vi "DAQAssistantTests.vi"() -> ()   [LabVIEW 2017]
panel:
  out "Numeric":dbl
  out "XY Graph":cluster{dbl[], dbl[]}(graph)
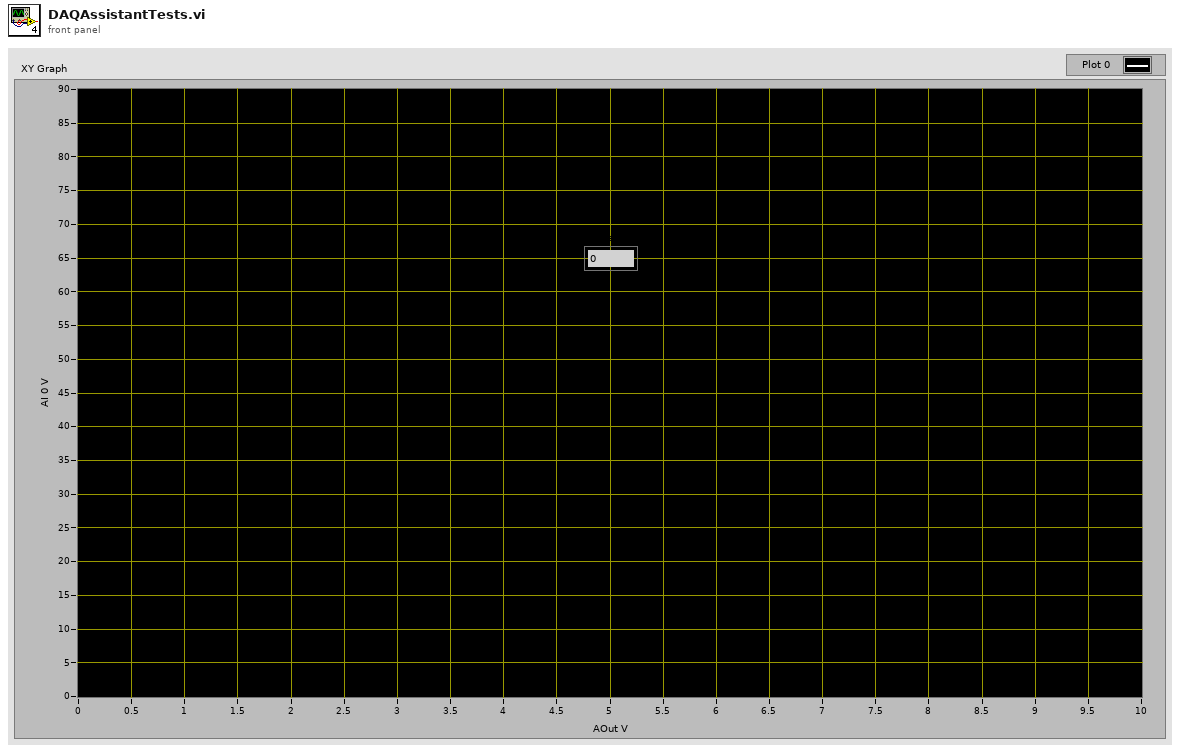
[diagram p1: front panel]
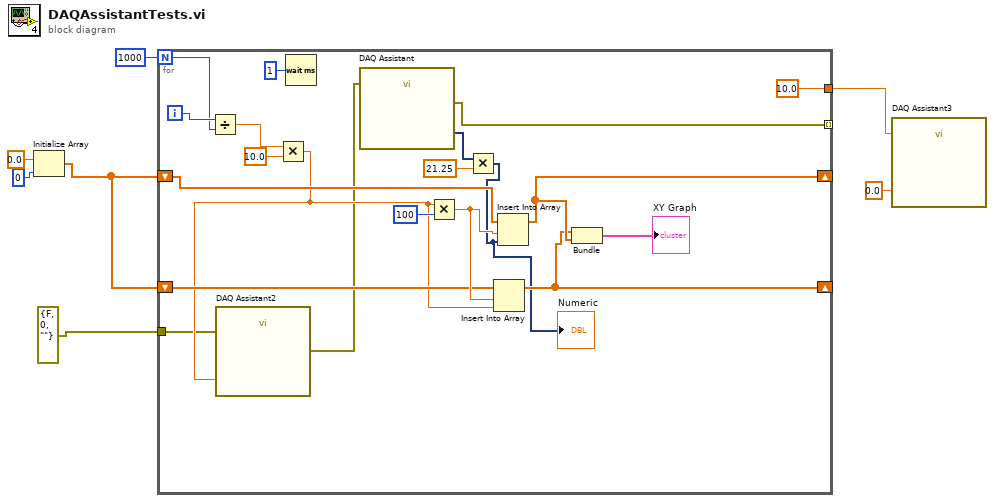
[diagram p0: block diagram]
diagram:
  n1 = Initialize Array(0.0 ("element"), 0 ("dimension size")) -> (w5:dbl[])
  n2 = for {
    N: 1000 -> [w18]
    shift-right: [w22] -> _
    shift-left: w5 -> [w27]
    shift-right: [w21] -> _
    shift-left: w5 -> [w24]
    tunnel: errorcluster {"status"=FALSE, "code"=0, "source"=""} ("error in") -> [w14]
    tunnel: [w12] -> _ mode=indexing
    tunnel: [10.0 ("timeout (s)")] -> w1
    i -> [w19]
    n3 = Divide(x=w19, y=w18) -> (x/y=w17:dbl)
    n4 = Multiply(x=w17, y=10.0) -> (x*y=w16:dbl)
    n5 = call "DAQ Assistant2"("data"=w16, "error in"=w14) -> ("error out"=w13:errorcluster)  [unwired: 16 in, 1 out]
    n6 = Wait (ms)(milliseconds to wait=u32 1) -> ()  [unwired: 1 out]
    n7 = call "DAQ Assistant"("error in"=w13) -> ("data"=w10:dynamicdata, "error out"=w12:errorcluster)  [unwired: 16 in, 1 out]
    n8 = Multiply(x=w16, y=100) -> (x*y=w25:dbl)
    n9 = Multiply(x=w10, y=21.25) -> (x*y=w8:dynamicdata)
    "Numeric" <- w8
    n10 = Insert Into Array(array=w24, index=w25, new element=w16) -> (w21:dbl[])
    n11 = Insert Into Array(array=w27, index=w25, new element=w8) -> (w22:dbl[])
    n12 = Bundle(w21, w22) -> (→"XY Graph":cluster{dbl[], dbl[]})  [unwired: 1 in]
  }
  n13 = call "DAQ Assistant3"("data"=0.0, "timeout (s)"=w1) -> ()  [unwired: 16 in, 2 out]
